vi "Write Single Register.vi"(8 "error in (no error)":errorcluster, 9 "value":u16, 10 "address":u16, 11 "MB session in":refnum<class "MB_Master.lvclass">) -> (0 "error out":errorcluster, 3 "MB session out":refnum<class "MB_Master.lvclass">)   [LabVIEW 2012, in "MB Master.lvlib"]
doc: "Function Code 6: Write <b>value</b> to holding register at <b>address</b>"
uses:
  MB Master.lvlib
  MB_Master.lvclass
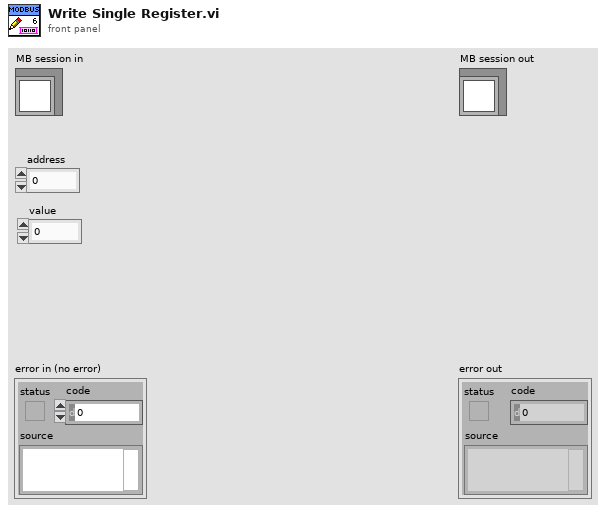
[diagram p1: front panel]
types:
  T1 = typedef "MB Master.lvlib/MB_PDU_Cluster.ctl" = cluster{"Function Code":u8, "Data":u8[], "RTU_DataBytes":u32}
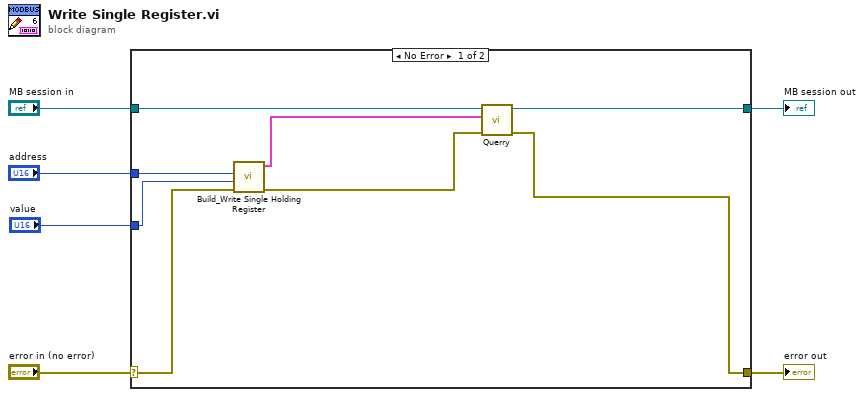
[diagram p0: block diagram]
diagram:
  n1 = case shown="No Error" "error in (no error)" {
    selector: "error in (no error)" -> [w11 w16]
    tunnel: [w10 w16] -> w5
    tunnel: [w13 w15] -> w3
    tunnel: "MB session in" -> [w8 w15]
    tunnel: "address" -> [w14 _]
    tunnel: "value" -> [w9 _]
    frame No Error {
      n2 = call "Build_Write Single Holding Register.vi"("error in (no error)"=w11, "value"=w9, "address"=w14) -> ("error out"=w12:errorcluster, "MB_PDU"=w7:T1)  [unwired: 7 in]
      n3 = call-dynamic "Querry.vi"("error in (no error)"=w12, "PDU_req"=w7, "MB_Master in"=w8) -> ("error out"=w10:errorcluster, "MB_Master out"=w13:refnum<class "MB_Master.lvclass">)  [unwired: 6 in, 1 out]
    }
    frame Error {
    }
  }
  "error out" <- w5
  "MB session out" <- w3
